vi "Get Pci Delay Generator.vi"(8 "error in (no error)":errorcluster) -> (0 "error out":errorcluster, 1 "Master":bool, 2 "Slot Number":i32, 3 "DG Product":i32(ring) items=["SRS_DG135"=1, "BME_DP01"=2, "BME_G02V3"=3, "BME_SG02V4"=4, "BME_G04"=5, "BME_G02V1"=6, "BME_G02V2"=7, "BME_SG02V1"=8, "BME_SG02V2"=9, "BME_SG02V3"=10, "BME_G03V1"=11, "BME_G03V2"=12, "BME_SG02V5"=13, "BME_G03V3"=14, "BME_G03V4"=15, "BME_SG02V6"=16, "BME_G03V5"=17, "BME_G05V1"=18, "BME_G05V2"=19, "BME_G05V3"=20, "BME_SG02V7"=21, "BME_SG02P1"=31, "BME_G03P1"=32, "BME_G05P1"=33, "BME_SG02P2"=34, "BME_G03P2"=35, "BME_SG02P3"=36, "BME_SG05P1"=37, "BME_G05P2"=38, "BME_SG05P2"=39, "BME_G05P3"=40, "BME_SG02P4"=41, "BME_SG02P5"=42, "BME_SG05P3"=43, "BME_SG08P1"=44], 5 "DG Number":i32)   [LabVIEW 2009, in "POLARIS BME DG.lvlib"]
doc: "long GetPciDelayGenerator(long* p_DG_Product, long* p_SlotNumber, BOOL* p_Master, long DG_Number);"
uses:
  POLARIS BME DG.lvlib
  BME DLL/DelayGenerator.dll
panel:
  # "NOTICE -- YOU MUST LEAVE THIS NOTICE IN PLACE.  PER THE TERMS OF THE LICENSE BELOW, YOU MAY SUBLICENSE THIS SOFTWARE \nIN ANY WAY THAT DOES NOT CONFLICT WITH THIS LICENSE.\n\n### BSD License (http://www.opensource.org/licenses/bsd-license.php) Begin ###\n \nCopyright (c) 2011, Applied Energetics, http://www.appliedenergetics.com,\n                               Richard Schwerdtfeger, <rschwerdtfeger@appliedenergetics.com>\n\nAll rights reserved.\n\nRedistribution and use in source and binary forms, with or without modification, are permitted provided that the \nfollowing conditions are met:\n\n    * Redistributions of source code must retain the above copyright notice, this list of conditions and the following disclaimer.\n    * Redistributions in binary form must reproduce the above copyright notice, this list of conditions and the following disclaimer \n       in the documentation and/or other materials provided with the distribution.\n    * Neither the name of Richard Schwerdtfeger, Applied Energetics, Inc., nor the names of its contributors may be used to \n       endorse or promote products derived from this software without specific prior written permission.\n\nTHIS SOFTWARE IS PROVIDED BY THE COPYRIGHT HOLDERS AND CONTRIBUTORS \"AS IS\" AND ANY EXPRESS OR IMPLIED WARRANTIES, \nINCLUDING, BUT NOT LIMITED TO, THE IMPLIED WARRANTIES OF MERCHANTABILITY AND FITNESS FOR A PARTICULAR PURPOSE ARE \nDISCLAIMED. IN NO EVENT SHALL THE COPYRIGHT OWNER OR CONTRIBUTORS BE LIABLE FOR ANY DIRECT, INDIRECT, INCIDENTAL,\n SPECIAL, EXEMPLARY, OR CONSEQUENTIAL DAMAGES (INCLUDING, BUT NOT LIMITED TO, PROCUREMENT OF SUBSTITUTE GOODS OR \nSERVICES; LOSS OF USE, DATA, OR PROFITS; OR BUSINESS INTERRUPTION) HOWEVER CAUSED AND ON ANY THEORY OF LIABILITY, \nWHETHER IN CONTRACT, STRICT LIABILITY, OR TORT (INCLUDING NEGLIGENCE OR OTHERWISE) ARISING IN ANY WAY OUT OF THE USE \nOF THIS SOFTWARE, EVEN IF ADVISED OF THE POSSIBILITY OF SUCH DAMAGE.\n\n### BSD License End ###"
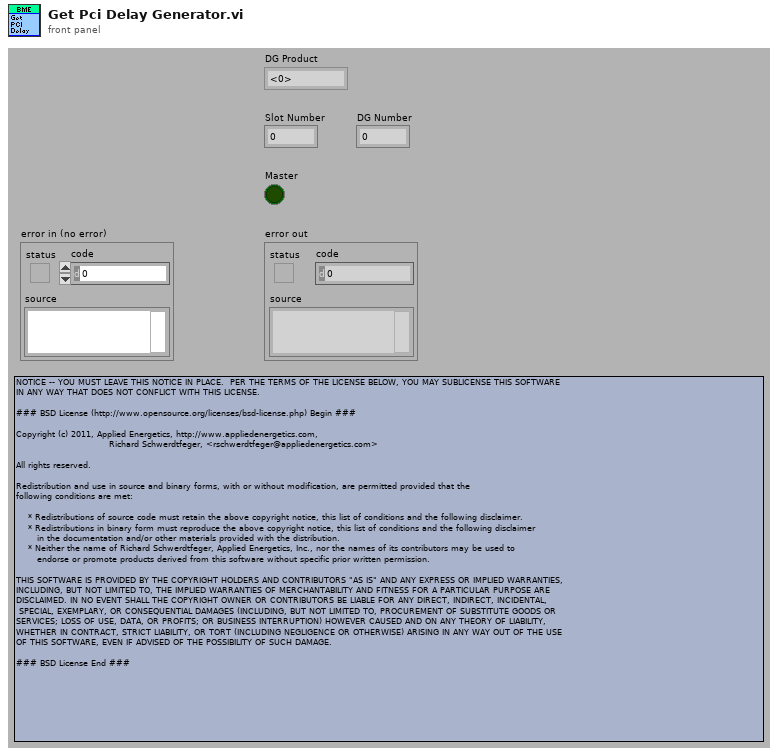
[diagram p1: front panel]
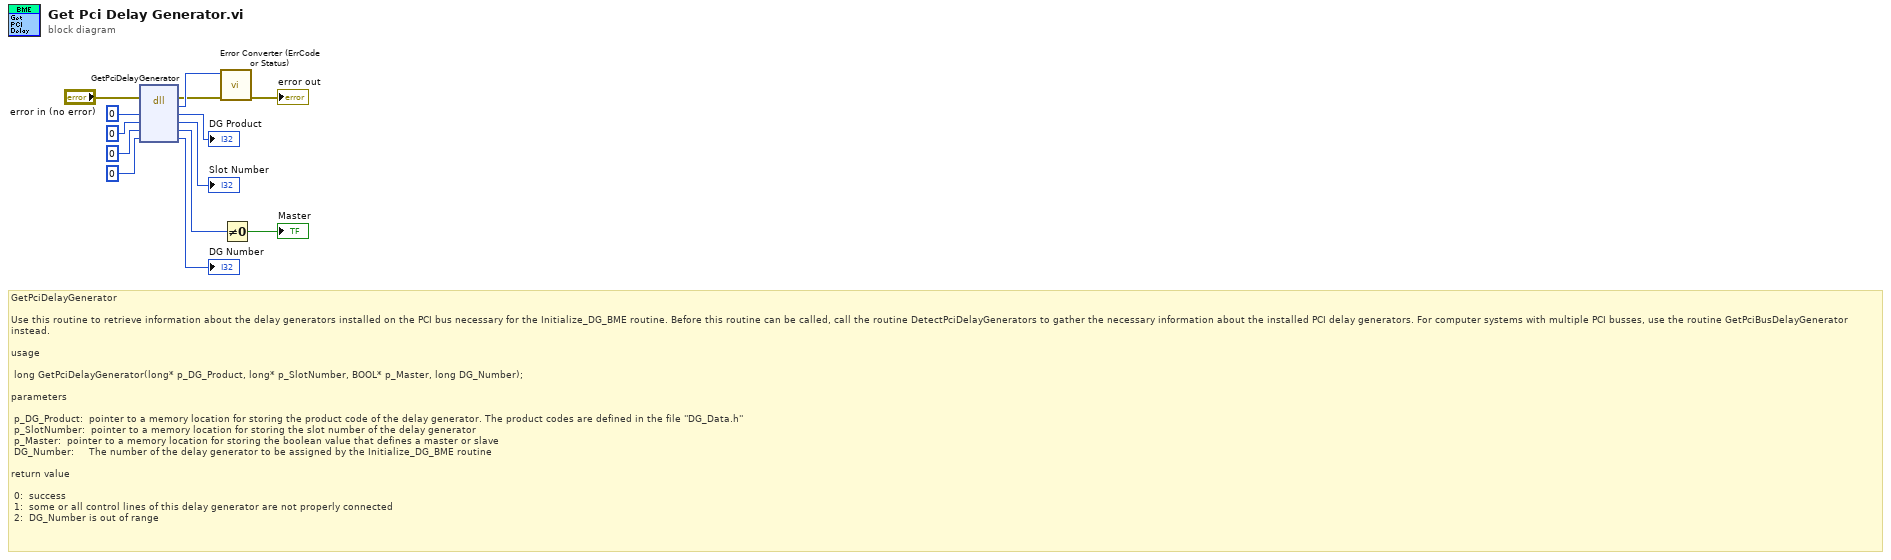
[diagram p0: block diagram]
diagram:
  # "GetPciDelayGenerator\n\nUse this routine to retrieve information about the delay generators installed on the PCI bus necessary for the Initialize_DG_BME routine. Before this routine can be called, call the routine DetectPciDelayGenerators to gather the necessary information about the installed PCI delay generators. For computer systems with multiple PCI busses, use the routine GetPciBusDelayGenerator instead.\n\nusage\n\n\tlong GetPciDelayGenerator(long* p_DG_Product, long* p_SlotNumber, BOOL* p_Master, long DG_Number);\n\nparameters\n\n\tp_DG_Product:\t\tpointer to a memory location for storing the product code of the delay generator. The product codes are defined in the file ''DG_Data.h''\n\tp_SlotNumber:\t\tpointer to a memory location for storing the slot number of the delay generator\n\tp_Master:\t\tpointer to a memory location for storing the boolean value that defines a master or slave\n\tDG_Number:   \t\tThe number of the delay generator to be assigned by the Initialize_DG_BME routine\n\nreturn value\n\n\t0:  success\n\t1:  some or all control lines of this delay generator are not properly connected\n\t2:  DG_Number is out of range"
  n1 = dll-call lib="C:/CS Framework/LVSCC/LV2009/GPL/Projects/cs-framework/CSClass/CSPOLARIS/POLARIS BME DG/BME DLL/DelayGenerator.*" fn="GetPciDelayGenerator"(error in="error in (no error)", "p_DG_Product"=0, "p_SlotNumber"=0, "p_Master"=0, "DG_Number"=0) -> (error out=w4:errorcluster, w13:i32, "p_DG_Product"=→"DG Product":i32, "p_SlotNumber"=→"Slot Number":i32, "p_Master"=w7:i32, "DG_Number"=→"DG Number":i32)  [unwired: 2 in, 1 out]
  n2 = call "Error Converter (ErrCode or Status).vi"("error in (no error)"=w4, "error code"=w13) -> ("error out"=→"error out":errorcluster)  [unwired: 9 out]
  n3 = Not Equal To 0?(x=w7) -> (x != 0?=→"Master":bool)
